vi "Init_Arduino.vi"(2 "error in (no error)":errorcluster, 3 "Velocidad de Conexion":enum16{"115200", "9600"}(ring), 4 "VISA Refnum in":refnum<visa-resource-name>) -> (0 "error out":errorcluster, 1 "VISA Refnum out":refnum<visa-resource-name>)   [LabVIEW 2014]
uses:
  <vilib>/Instr/_visa.llb/VISA Find Search Mode.ctl
  <vilib>/Instr/_visa.llb/VISA Configure Serial Port (Instr).vi
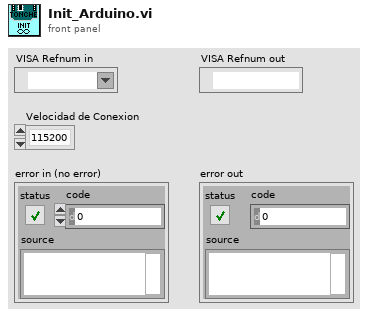
[diagram p1: front panel]
types:
  T1 = typedef "VISA Find Search Mode.ctl" = u32
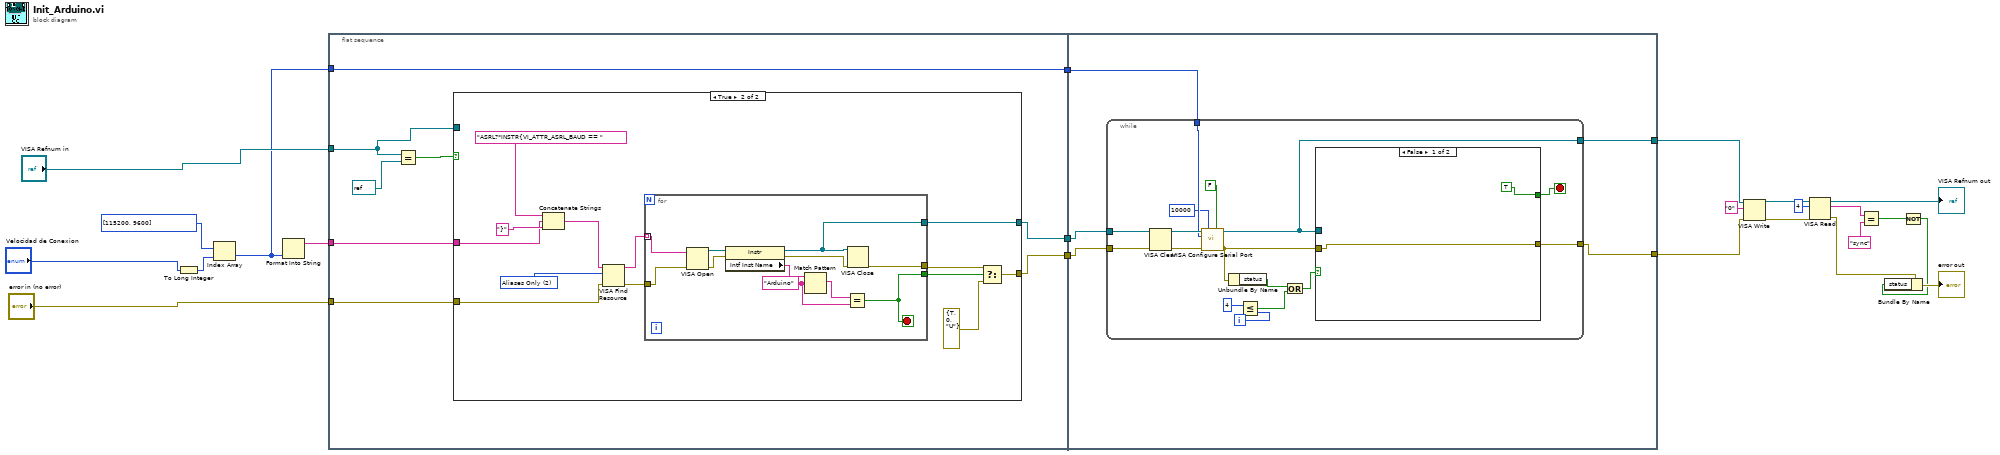
[diagram p0: block diagram]
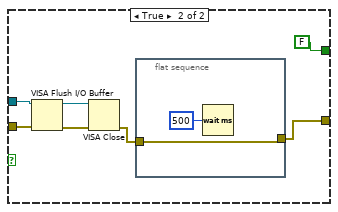
[diagram p3: hidden frame]
diagram:
  n1 = To Long Integer(number="Velocidad de Conexion") -> (32bit integer=w3:i32)
  n2 = Index Array(array=i32[] [115200, 9600], index=w3) -> (element=w17:i32)
  n3 = Format Into String(w17) -> (resulting string=w5:string)  [unwired: 3 in, 1 out]
  n4 = flat-sequence {
    tunnel: "VISA Refnum in" -> [w29]
    tunnel: "error in (no error)" -> [w28]
    tunnel: w5 -> [w27]
    tunnel: w17 -> [w24]
    tunnel: [w26] -> w23
    tunnel: [w25] -> w22
    tunnel: [w24] -> w21
    tunnel: w23 -> [w60]
    tunnel: w22 -> [w61]
    tunnel: w21 -> [w62]
    tunnel: [w59] -> w18
    tunnel: [w58] -> w19
    frame #0 {
      n5 = Equal?(x=w29, y=refnum<visa-resource-name> refnum ("VISA resource name 2")) -> (x = y?=w30:bool)
      n6 = case shown="True" w30 {
        tunnel: [w33 w37] -> w25
        tunnel: w29 -> [w32 _]
        tunnel: w28 -> [w33 w36]
        tunnel: [w32 w35] -> w26
        tunnel: w27 -> [_ w34]
        frame False {
        }
        frame True {
          w46 = T1 2 items=["Canonical Names Only"=0, "Aliases Only"=2, "Include Matching Aliases"=3, "Include All Aliases"=4] ("Search Mode")
          n7 = Concatenate Strings("ASRL?*INSTR{VI_ATTR_ASRL_BAUD == " ("string"), w34, "}" ("string")) -> (w41:string)
          n8 = VISA Find Resource(8:w36, 10:w46, 11:w41) -> (0:w44:errorcluster, 3:w45:string[])  [unwired: 1 out]
          n9 = for {
            tunnel: w45 -> [w56] mode=indexing
            tunnel: w44 -> [w57]
            tunnel: [w50] -> w35
            tunnel: [w48] -> w40
            tunnel: [w47] -> w38
            stop <- w47 stop-if-true
            w51 = "Arduino" ("regular expression")
            n10 = VISA Open(error in (no error)=w57, VISA resource name=w56) -> (VISA resource name=w55:refnum<visa-resource-name>, error out=w54:errorcluster)  [unwired: 3 in]
            n11 = property class="Instr"(reference=w55, error in=w54) -> (reference out=w50:refnum<visa-resource-name>, error out=w49:errorcluster, "Intf Inst Name"=w53:string)
            n12 = Match Pattern(string=w53, regular expression=w51) -> (match substring=w52:string)  [unwired: 1 in, 3 out]
            n13 = Equal?(x=w52, y=w51) -> (x = y?=w47:bool)
            n14 = VISA Close(VISA resource name=w50, error in (no error)=w49) -> (error out=w48:errorcluster)
          }
          n15 = Select(t=w40, s=w38, f=errorcluster {"status"=TRUE, "code"=0, "source"="U"} ("error out")) -> (s? t:f=w37:errorcluster)
        }
      }
    }
    frame #1 {
      n16 = while {
        tunnel: w62 -> [w76]
        tunnel: w60 -> [w73]
        tunnel: w61 -> [w72]
        tunnel: [w64] -> w58
        tunnel: [w63] -> w59
        i -> [w70]
        stop <- w65 stop-if-true
        n17 = VISA Clear(VISA resource name=w73, error in (no error)=w72) -> (VISA resource name out=w78:refnum<visa-resource-name>, error out=w77:errorcluster)
        n18 = call-poly "VISA Configure Serial Port"("VISA resource name"=w78, "timeout (10sec)"=u32 10000, "Enable Termination\nChar (T)"=FALSE ("Enable Termination\nChar (T)"), "baud rate (9600)"=w76, "error in (no error)"=w77) -> ("VISA resource name out"=w63:refnum<visa-resource-name>, "error out"=w66:errorcluster)  [unwired: 9 in]
        n19 = Unbundle By Name(w66) -> ("status"=w71:bool)
        n20 = Less Or Equal?(x=4, y=w70) -> (x <= y?=w68:bool)
        n21 = Or(x=w71, y=w68) -> (x .or. y?=w67:bool)
        n22 = case shown="False" w67 {
          tunnel: w66 -> [w79 w87]
          tunnel: w63 -> [_ w86]
          tunnel: [TRUE FALSE] -> w65
          tunnel: [w79 w81] -> w64
          frame False {
          }
          frame True {
            n23 = VISA Flush I/O Buffer(VISA resource name=w86, error in (no error)=w87) -> (VISA resource name out=w84:refnum<visa-resource-name>, error out=w85:errorcluster)  [unwired: 1 in]
            n24 = VISA Close(VISA resource name=w84, error in (no error)=w85) -> (error out=w82:errorcluster)
            n25 = flat-sequence {
              tunnel: [w88] -> w81
              tunnel: w82 -> [w88]
              frame #0 {
                n26 = Wait (ms)(milliseconds to wait=u32 500) -> ()  [unwired: 1 out]
              }
            }
          }
        }
      }
    }
  }
  n27 = VISA Write(VISA resource name=w18, write buffer="0", error in (no error)=w19) -> (VISA resource name out=w7:refnum<visa-resource-name>, error out=w8:errorcluster)  [unwired: 1 out]
  n28 = VISA Read(VISA resource name=w7, byte count=u32 4, error in (no error)=w8) -> (VISA resource name out=→"VISA Refnum out":refnum<visa-resource-name>, read buffer=w9:string, error out=w11:errorcluster)  [unwired: 1 out]
  n29 = Equal?(x=w9, y="sync") -> (x = y?=w12:bool)
  n30 = Not(x=w12) -> (.not. x?=w13:bool)
  n31 = Bundle By Name(cluster=w11, "status"=w13) -> (→"error out":errorcluster)
